vi "DAQmx read position error fix.vi"(0 "task in":refnum<k21>, 1 "samples to read":i32, 2 "error in":errorcluster) -> (3 "task out":refnum<k21>, 4 "samples available":i32, 5 "position mode":i32, 6 "error out":errorcluster)   [LabVIEW 2012]
uses:
  <resource>/objmgr/daqmx.rc
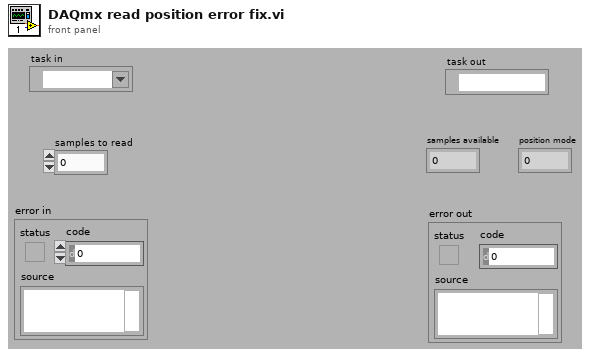
[diagram p1: front panel]
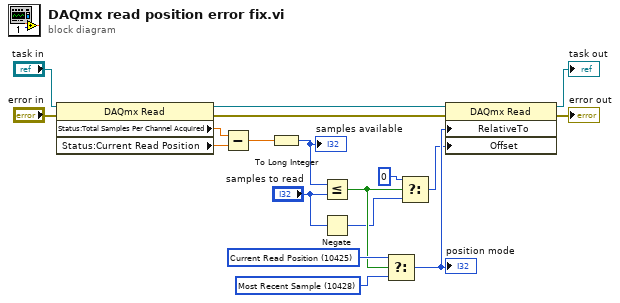
[diagram p0: block diagram]
diagram:
  w9 = 10425 items=["First Sample"=10424, "Current Read Position"=10425, "Reference Trigger"=10426, "First Pretrigger Sample"=10427, "Most Recent Sample"=10428] ("RelativeTo")
  w8 = 10428 items=["First Sample"=10424, "Current Read Position"=10425, "Reference Trigger"=10426, "First Pretrigger Sample"=10427, "Most Recent Sample"=10428] ("RelativeTo")
  n1 = property class="DAQmx Read"(reference="task in", error in="error in") -> (reference out=w15:refnum<k21>, error out=w13:errorcluster, "Status:Total Samples Per Channel Acquired"=w12:dbl, "Status:Current Read Position"=w11:dbl)
  n2 = Subtract(x=w12, y=w11) -> (x-y=w10:dbl)
  n3 = To Long Integer(number=w10) -> (32bit integer=w1:i32)
  "samples available" <- w1
  n4 = Less Or Equal?(x=w1, y="samples to read") -> (x <= y?=w5:bool)
  n5 = Negate(x="samples to read") -> (-x=w3:i32)
  n6 = Select(t=w9, s=w5, f=w8) -> (s? t:f=w7:i32)
  "position mode" <- w7
  n7 = Select(t=0, s=w5, f=w3) -> (s? t:f=w2:i32)
  n8 = property class="DAQmx Read"(reference=w15, error in=w13, "RelativeTo"=w7, "Offset"=w2) -> (reference out=→"task out":refnum<k21>, error out=→"error out":errorcluster)
